vi "Get Disable Symbol Value by VI.vi"(8 "error in (no error)":errorcluster, 10 "Disable Symbol":string, 11 "VI Refnum":refnum<vi>) -> (0 "error out":errorcluster, 1 "Found?":bool, 2 "Value":string)   [LabVIEW 2021, in "Personality.lvlib"]
doc: "Gets the specified disable symbol value from the specified VI reference."
uses:
  <vilib>/myRIO/Common/FPGA Personality Framework/Personality.lvlib
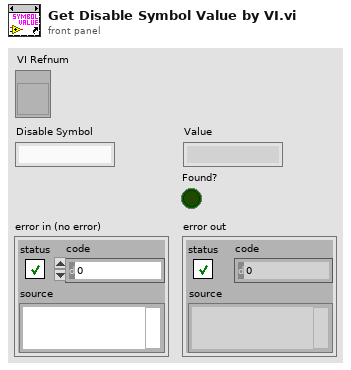
[diagram p1: front panel]
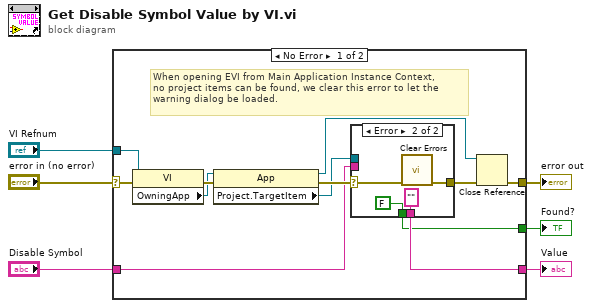
[diagram p0: block diagram]
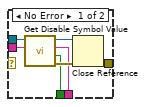
[diagram p2: hidden frame]
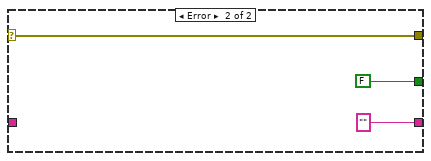
[diagram p3: hidden frame]
diagram:
  n1 = case shown="No Error" "error in (no error)" {
    selector: "error in (no error)" -> [w18 w32]
    tunnel: [w16 "" ("Value")] -> w5
    tunnel: [w15 FALSE ("Found?")] -> w4
    tunnel: "VI Refnum" -> [w14 _]
    tunnel: "Disable Symbol" -> [w7 _]
    tunnel: [w12 w32] -> w1
    frame No Error {
      # "When opening EVI from Main Application Instance Context,\nno project items can be found, we clear this error to let the \nwarning dialog be loaded."
      n2 = property class="VI"(reference=w14, error in=w18) -> (error out=w13:errorcluster, "OwningApp"=w10:refnum<vi>)  [unwired: 1 out]
      n3 = property class="App"(reference=w10, error in=w13) -> (reference out=w11:refnum<vi>, error out=w9:errorcluster, "Project.TargetItem"=w8:refnum<vi>)
      n4 = case shown="Error" w9 {
        selector: w9 -> [_ w27]
        tunnel: [w24 w28] -> w17
        tunnel: [w20 "" ("Value")] -> w16
        tunnel: [w19 FALSE ("Found?")] -> w15
        tunnel: w7 -> [w25 _]
        tunnel: w8 -> [w21 _]
        frame No Error {
          n5 = call <vilib>:"Get Disable Symbol Value.vi"("Disable Symbol"=w25, "TargetItem Refnum"=w21) -> ("error out"=w23:errorcluster, "Found?"=w19:bool, "Value"=w20:string, "Duplicated TargetItem Refnum"=w22:refnum<vi>)  [unwired: 6 in]
          n6 = Close Reference(reference=w22, error in (no error)=w23) -> (error out=w24:errorcluster)
        }
        frame Error {
          n7 = call <vilib>:"Clear Errors.vi"("error in (no error)"=w27) -> ("error out"=w28:errorcluster)  [unwired: 5 in, 1 out]
        }
      }
      n8 = Close Reference(reference=w11, error in (no error)=w17) -> (error out=w12:errorcluster)
    }
    frame Error {
    }
  }
  "Value" <- w5
  "error out" <- w1
  "Found?" <- w4
